vi "Read StartPos.vi"(8 "error in (no error)":errorcluster, 11 "PongPanel in":refnum<class "PongPanel.lvclass">) -> (0 "error out":errorcluster, 2 "Coordinate":T1, 3 "PongPanel out":refnum<class "PongPanel.lvclass">)   [LabVIEW 2019, in "RT_Game.lvlib" / "PongPanel.lvclass"]
uses:
  PongPanel.lvclass
  Game/Coordinate.ctl
  PongPanel.lvclass/PongPanel.ctl
  Game/Game.lvclass
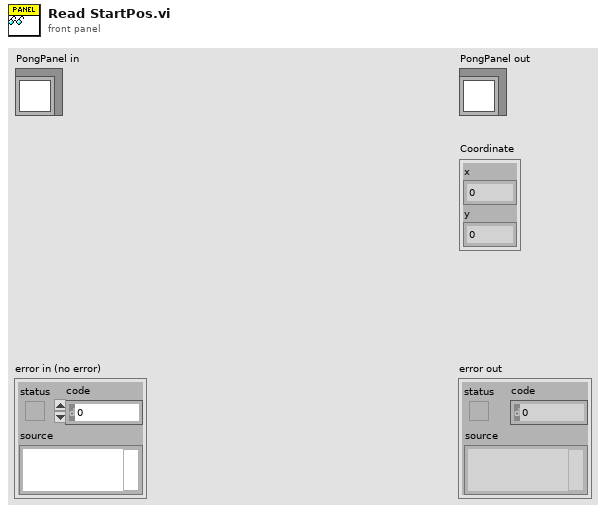
[diagram p1: front panel]
types:
  T1 = typedef "RT_Game.lvlib/Game.lvclass/Coordinate.ctl" = cluster{"x":dbl, "y":dbl}
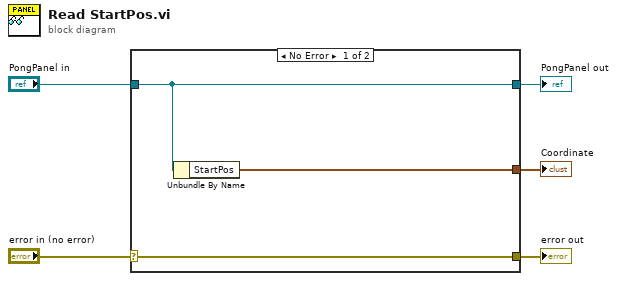
[diagram p0: block diagram]
diagram:
  n1 = case shown="No Error" "error in (no error)" {
    selector: "error in (no error)" -> [w8 w9]
    tunnel: [w8 w9] -> w4
    tunnel: [w7 w10] -> w2
    tunnel: "PongPanel in" -> [w7 w10]
    tunnel: [w6 _] -> w1
    frame No Error {
      n2 = Unbundle By Name(w7) -> ("StartPos"=w6:T1)
    }
    frame Error {
    }
  }
  "error out" <- w4
  "PongPanel out" <- w2
  "Coordinate" <- w1
